vi "IMU Main.vi"() -> ()   [LabVIEW 2021]
doc: "This Continuous Measurement sample project is based on the Queued Message Handler template.\n\nThe Event Handling Loop generates messages based on user interface actions.\n\nThe Message Handling Loop processes messages generated by the Event Handling Loop, or by other messages. There are also Acquisition and Logging message handling loop subVIs, and a chart updating loop."
uses:
  Acquisition/IMU Data Queue.ctl
  IMU TimeDataStruct.ctl
  Acquisition/IMU Data Notifier.ctl
  Settings/Settings.ctl
  Acquisition/Hardware Configuration.ctl
  Settings/baudrates.ctl
  Logging/Logging Configuration.ctl
  controls/IMU UI Data.ctl
  controls/IMU UI State.ctl
  <vilib>/Platform/TimedLoop/XDataNode/timing_clust.ctl
  <vilib>/Platform/TimedLoop/XDataNode/nitl_modes.ctl
  <vilib>/Platform/TimedLoop/XDataNode/wakeup.ctl
  support/Message Queue/Enqueue Message (Single).vi
  support/Message Queue/Enqueue Message (Array).vi
  <vilib>/Utility/error.llb/Error Cluster From Error Code.vi
  <vilib>/ErrorRing/Error Ring.xnode
  <vilib>/platform/TimedLoop/XDataNode/XDataNode.xnode
  Acquisition/IMU Acquisition.lvlib
  Settings/IMU Settings.lvlib
  Logging/IMU Logging.lvlib
  support/User Event - Stop/IMU User Event - Stop.lvlib
  support/Message Queue/IMU Message Queue.lvlib
  Settings/Settings Dialog.vi
  Processing/IMU Processing.lvlib
  <vilib>/Platform/TimedLoop/XDataNode/XDNodeRunTimeDep.lvlib
  <vilib>/picture/3D Picture Control/NI_3D Picture Control.lvlib
  Processing/QuaternionLibrary/QuaternionLibrary.lvlib
panel:
  out "Quaternion":dbl[](array[numeric])
  out "IMU":refnum<vi>(3d-picture)
  in  "Enum 3":enum16{"None", "Disc", "Box", "STL"}(ring)=enum."Disc"
  in  "Frequency":i64
  in  "Data Queue Processing":T1
  in  "Data Notifier":T2
  in  "Data Queue Logging":T1
  in  "Settings":bool
  in  "Start":bool
  in  "Stop":bool
  out "Status":string
  in  "Exit":bool
  # "Continuous Measurement Data Logger"
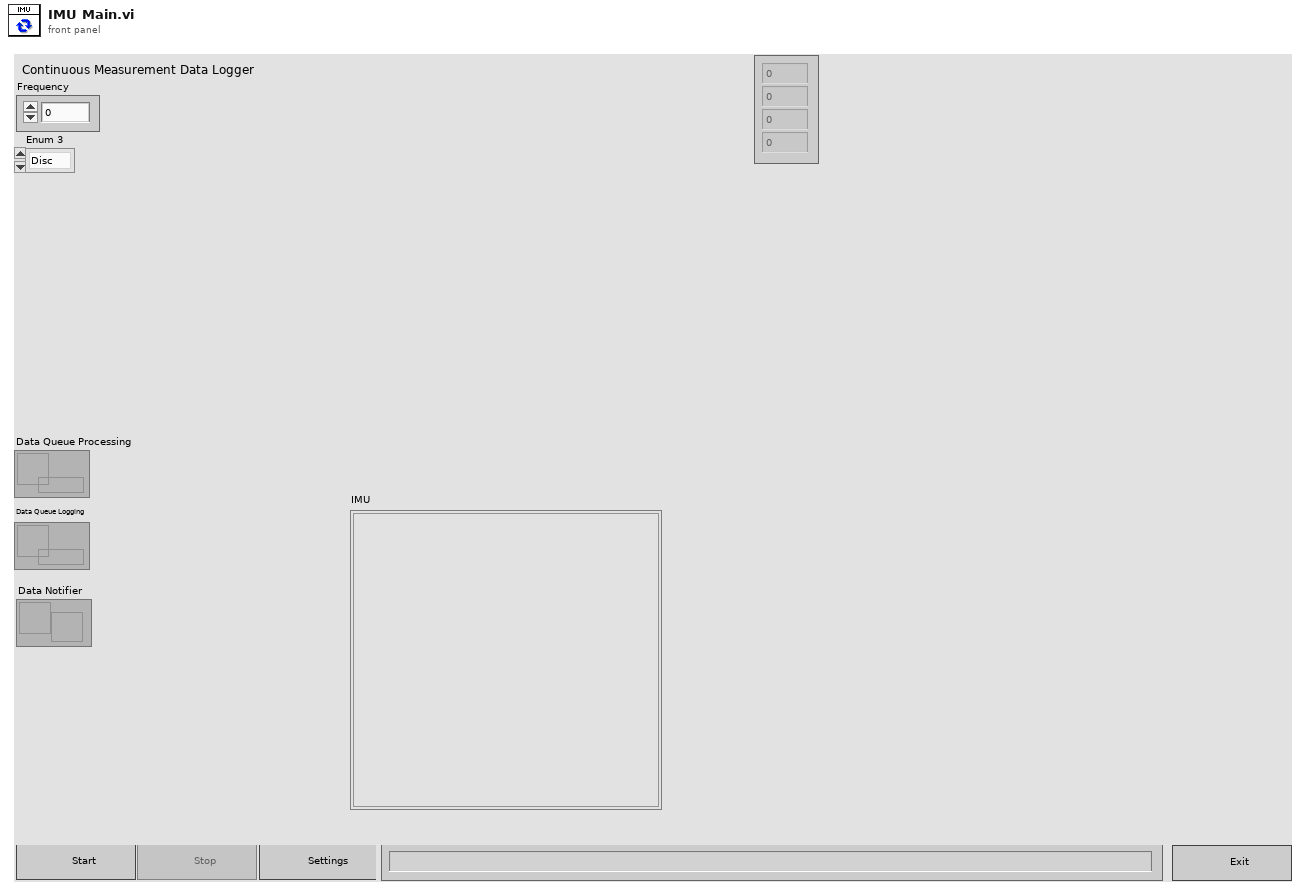
[diagram p1: front panel]
types:
  T1 = typedef "IMU Data Queue.ctl" = refnum<queue>
  T2 = typedef "IMU Data Notifier.ctl" = refnum<notifier>
  T3 = typedef "IMU TimeDataStruct.ctl" = cluster{string, dbl[]}
  T4 = typedef "IMU UI State.ctl" = enum16{"Idle", "Acquiring and Logging", "Waiting for Exit", "Waiting for Exit (Acq Stopped)", "Waiting for Exit (Log Stopped)", "Waiting for Stop", "Waiting for Stop (Acq Stopped)", "Waiting for Stop (Log Stopped)"}
  T5 = typedef "IMU UI Data.ctl" = cluster{"Start Ref":refnum<vi>, "Stop Ref":refnum<vi>, "Settings Ref":refnum<vi>, "Exit Ref":refnum<vi>, "Status Ref":refnum<vi>}
  T6 = typedef "IMU Settings.lvlib/Settings.ctl" = cluster{"Hardware Configuration":T7, "Logging Configuration":T9}
  T7 = typedef "IMU Acquisition.lvlib/Hardware Configuration.ctl" = cluster{"Port":refnum<visa-resource-name>, "Baudrate":T8}
  T8 = typedef "baudrates.ctl" = u16
  T9 = typedef "IMU Logging.lvlib/Logging Configuration.ctl" = cluster{"Log File Base Path":path, "TDMS File Reference":refnum<k34>, "Log Select":bool}
  T10 = typedef "IMU Message Queue.lvlib/All Message Queues.ctl" = cluster{"UI":refnum<queue>, "Acquisition":refnum<queue>, "Logging":refnum<queue>, "Processing":refnum<queue>}
  T11 = typedef "XDNodeRunTimeDep.lvlib/timing_clust.ctl" = cluster{"Expected End [f-1]":u64, "Actual End [f-1]":u64, "Finished Late? [f-1]":bool, "Expected End [i-1]":u64, "Actual End [i-1]":u64, "Finished Late? [i-1]":bool, "Expected Start [i]":u64, "Actual Start [i]":u64, "Expected Start [f]":u64, "Actual Start [f]":u64, "Source Name":string, "Structure Name":string, "Period":i64, "Deadline":i64, "Offset":i64, "Start":i64, "Priority":i32, "Timeout":i32, "Mode":T12, "Wakeup Reason":T13, "Error":errorcluster, "Source Type":string, "Secondary Source Type":string, "Global End Time":u64, "Global Start Time":u64, "Frame Duration":u64, "Iteration Duration":u64, "Assigned CPU":i32, "I/O Scan Engine Mode":u32}
  T12 = typedef "XDNodeRunTimeDep.lvlib/nitl_modes.ctl" = enum32{"No Change", "Process missed periods, maintain original phase", "Discard missed periods, maintain original phase", "Process missed periods, ignore original phase", "Discard missed periods, ignore original phase"}
  T13 = typedef "XDNodeRunTimeDep.lvlib/wakeup.ctl" = enum32{"Normal", "Aborted", "Asynchronous wakeup", "Timing source error", "Timed loop error", "Timeout"}
  T14 = cluster{"axis[0]":dbl, "axis[1]":dbl, "axis[2]":dbl}
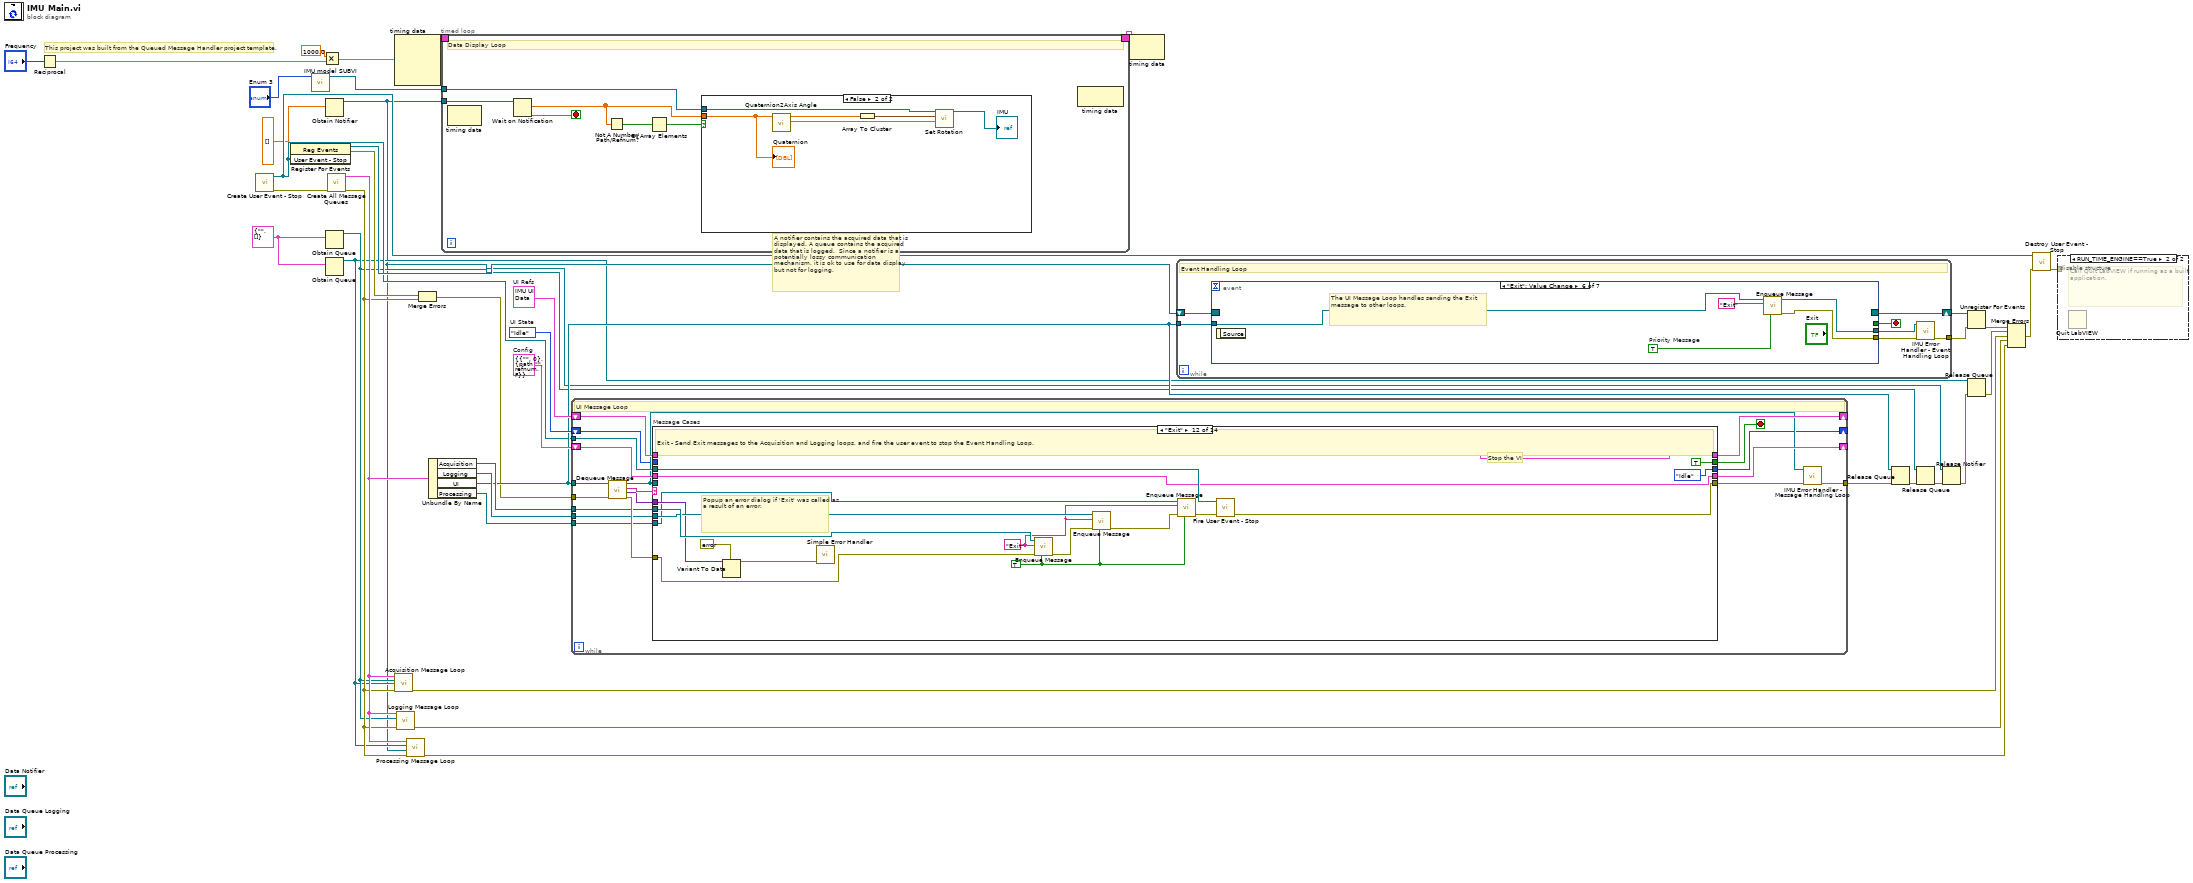
[diagram p0: block diagram]
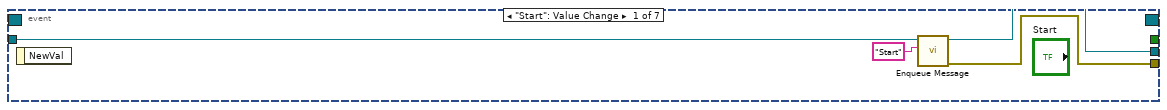
[diagram p4: hidden frame]
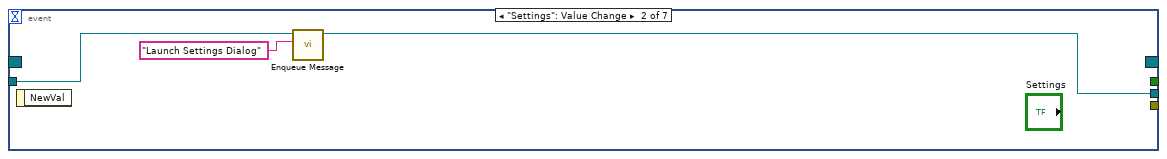
[diagram p5: hidden frame]
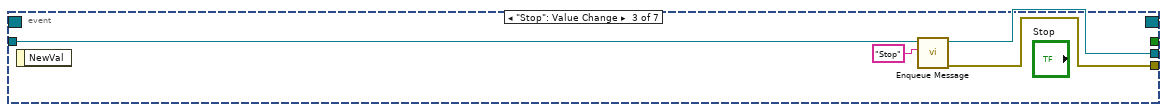
[diagram p6: hidden frame]
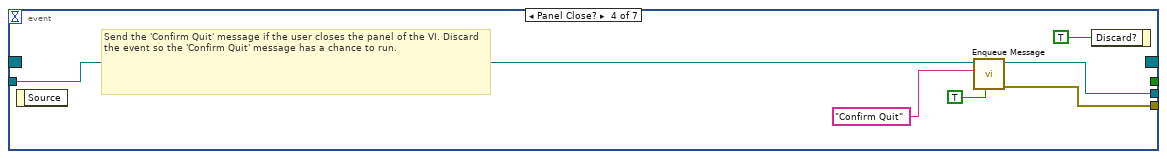
[diagram p7: hidden frame]
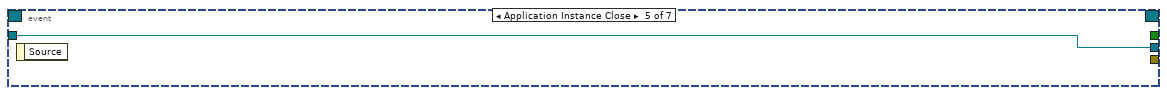
[diagram p8: hidden frame]
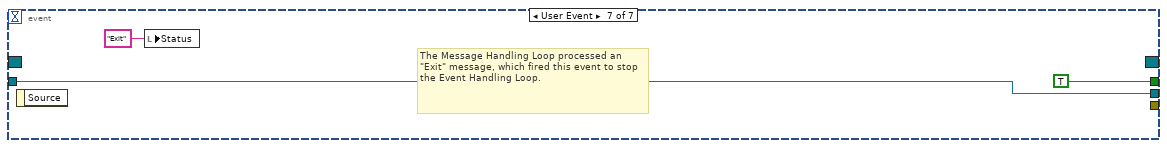
[diagram p9: hidden frame]
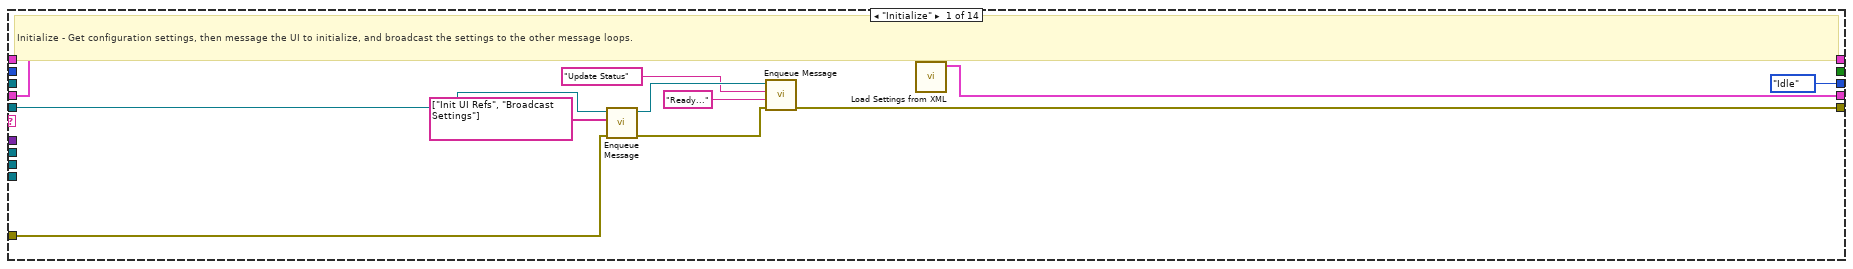
[diagram p10: hidden frame]
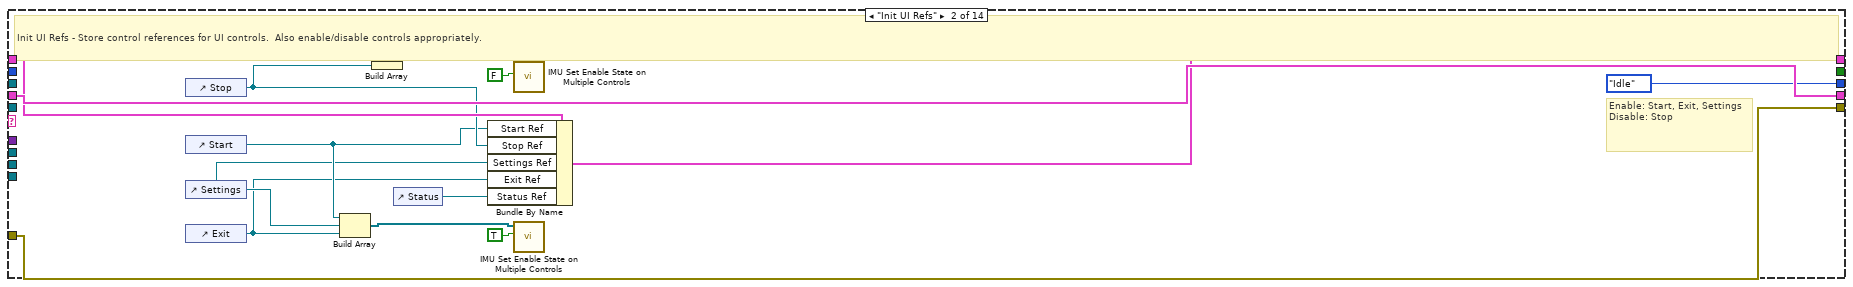
[diagram p11: hidden frame]
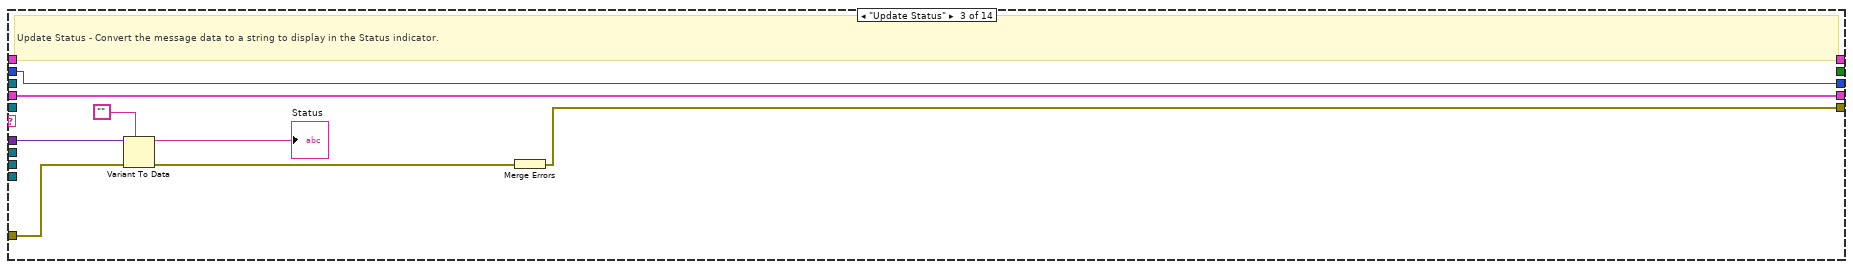
[diagram p12: hidden frame]
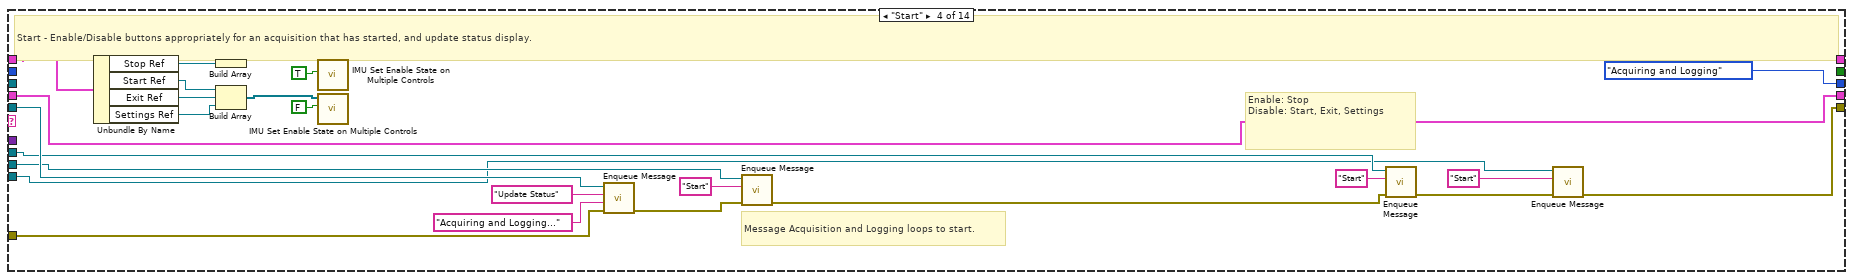
[diagram p13: hidden frame]
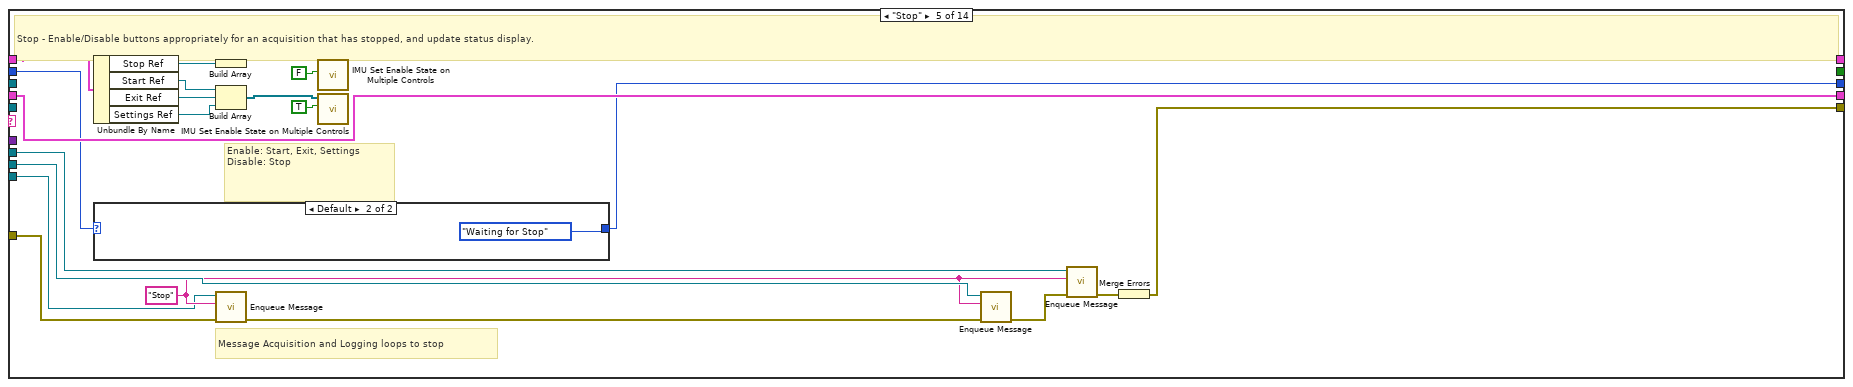
[diagram p14: hidden frame]
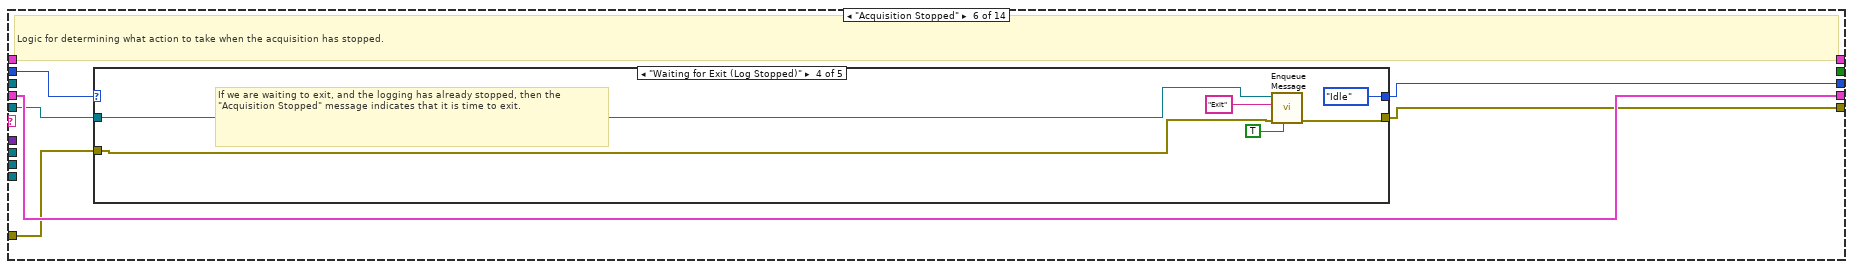
[diagram p16: hidden frame]
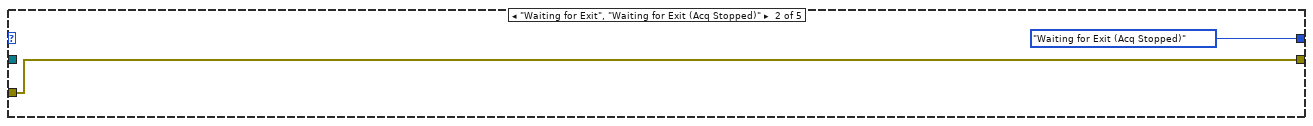
[diagram p18: hidden frame]
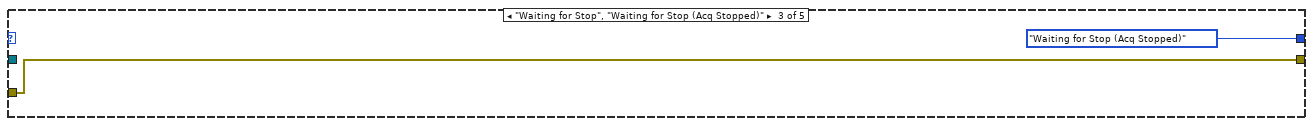
[diagram p19: hidden frame]
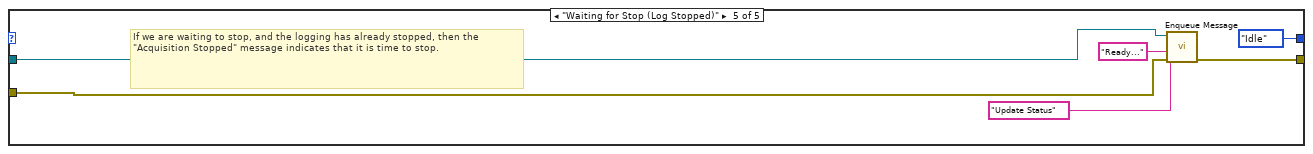
[diagram p20: hidden frame]
diagram:
  w19 = T3 {"", []}
  w29 = IMU_UI_State."Idle"  # UI State
  w32 = T5 {"Start Ref"=refnum, "Stop Ref"=refnum, "Settings Ref"=refnum, "Exit Ref"=refnum, "Status Ref"=refnum}  # UI Refs
  w35 = T6 {"Hardware Configuration"={"Port"="", "Baudrate"=0}, "Logging Configuration"={"Log File Base Path"=path "", "TDMS File Reference"=refnum, "Log Select"=FALSE}}  # Config
  # "This project was built from the Queued Message Handler project template."
  n1 = Reciprocal(x="Frequency") -> (1/x=w9:dbl)
  n2 = call "Create User Event - Stop.vi"() -> ("error out"=w37:errorcluster, "User Event - Stop"=w22:refnum<user-event>)  [unwired: 10 in]
  n3 = register-events(w22) -> (reference out=w23:refnum<event-registration>, error out=w20:errorcluster)  [unwired: 2 in]
  n4 = call "IMU model SUBVI.vi"("Enum 3"="Enum 3") -> ("SceneObject out"=w3:refnum<vi>)  [unwired: 10 in]
  n5 = Multiply(x=1000.0, y=w9) -> (x*y=w1:dbl)
  n6 = Obtain Queue(element data type=w19) -> (queue out=w14:refnum<queue>)  [unwired: 4 in, 2 out]
  n7 = Obtain Queue(element data type=w19) -> (queue out=w13:refnum<queue>)  [unwired: 4 in, 2 out]
  n8 = Obtain Notifier(notification data type=dbl[] []) -> (notifier out=w2:refnum<notifier>)  [unwired: 3 in, 2 out]
  n9 = call "Create All Message Queues.vi"("error in (no error)"=w37) -> ("error out"=w16:errorcluster, "Message Queues out"=w17:T10)  [unwired: 9 in]
  n10 = node-c288(w1) -> (w5:T11)  [unwired: 3 in]
  n11 = call "Acquisition Message Loop.vi"("Message Queues"=w17, "Data Queue Logging"=w14, "Data Queue Processing"=w13, "error in (no error)"=w16) -> ("error out"=w38:errorcluster)  [unwired: 11 in]
  n12 = call "Logging Message Loop.vi"("error in (no error)"=w16, "Data Queue"=w14, "Message Queues"=w17) -> ("error out"=w36:errorcluster)  [unwired: 8 in]
  n13 = call "Processing Message Loop.vi"("error in (no error)"=w16, "Data Notifier"=w2, "Data Queue"=w13, "Message Queues"=w17) -> ("error out"=w15:errorcluster)  [unwired: 7 in]
  n14 = Merge Errors(w20, w16) -> (w21:errorcluster)
  n15 = Unbundle By Name(w17) -> ("Acquisition"=w31:refnum<queue>, "Logging"=w30:refnum<queue>, "UI"=w27:refnum<queue>, "Processing"=w18:refnum<queue>)
  n16 = timed-loop "Data Display Loop" {
    timing: w5 -> [_]
    timing-out: [_] -> w4
    tunnel: w3 -> [w44]
    tunnel: w2 -> [w45]
    stop <- w46 stop-if-true
    # "A notifier contains the acquired data that is displayed. A queue contains the acquired data that is logged.  Since a notifier is a potentially lossy communication mechanism, it is ok to use for data display, but not for logging."
    # "Data Display Loop"
    n17 = node-c288() -> ()  [unwired: 1 in, 1 out]
    n18 = Wait on Notification(notifier=w45) -> (notification=w42:dbl[], error out=w46:errorcluster)  [unwired: 3 in, 2 out]
    n19 = Not A Number/Path/Refnum?(number/path/refnum=w42) -> (NaN/Path/Refnum?=w41:bool[])
    n20 = Or Array Elements(Boolean array=w41) -> (logical OR=w43:bool)
    n21 = case shown="False" w43 {
      tunnel: w42 -> [_ w52]
      tunnel: w44 -> [_ w48]
      frame True {
      }
      frame False {
        n22 = call <userlib>:"Quaternion2Axis Angle.vi"("quaternion"=w52) -> ("angle"=w51:sgl, "axis"=w50:dbl[])  [unwired: 8 in, 1 out]
        n23 = Array To Cluster(array=w50) -> (cluster=w49:T14)
        n24 = call <vilib>:"Set Rotation.vi"("Angle"=w51, "Axis"=w49, "Scene Object"=w48) -> ("Rotated Scene Object"=→"IMU":refnum<vi>)  [unwired: 7 in, 1 out]
        "Quaternion" <- w52
      }
    }
    n25 = node-c288() -> ()  [unwired: 1 in, 1 out]
  }
  n26 = while {
    tunnel: w27 -> [w67]
    tunnel: w22 -> [w72]
    shift-right: [w66] -> _
    shift-left: w35 -> [w65]
    shift-right: [w63] -> _
    shift-left: w32 -> [w64]
    tunnel: w31 -> [w62]
    tunnel: w30 -> [w61]
    shift-right: [w56] -> _
    shift-left: w29 -> [w57]
    tunnel: w21 -> [w71]
    tunnel: [w60] -> w40
    tunnel: w18 -> [w55]
    stop <- w73 stop-if-true
    # "UI Message Loop"
    n27 = call "Dequeue Message.vi"("error in (no error)"=w71, "Message Queue"=w67) -> ("error out"=w70:errorcluster, "Message Data"=w68:variant, "Message"=w69:string, "dup Message Queue"=w58:refnum<queue>)  [unwired: 6 in]
    n28 = case "Message Cases" shown="\"Exit\"" w69 {
      selector: w69 -> [_ _ _ _ _ _ _ _ _ _ _ _ _ w294]
      tunnel: w58 -> [w77 _ _ w133 _ w159 w184 _ w224 _ w245 _ _ _]
      tunnel: w70 -> [w76 w99 w107 w132 w136 w160 w185 w213 w226 w233 w244 w278 w292 _]
      tunnel: [w81 w99 w108 w110 w154 w157 w182 w218 w219 w236 w243 w285 w291 w293] -> w59
      tunnel: [_ _ _ _ _ _ _ _ _ _ _ TRUE _ _] -> w73
      tunnel: w68 -> [_ _ w106 _ _ _ _ _ _ w237 _ w276 _ _]
      tunnel: w72 -> [_ _ _ _ _ _ _ _ _ _ _ w286 _ _]
      tunnel: [w84 w98 w102 w131 w153 w163 w188 w216 w223 w241 w248 w284 w290 w297] -> w66
      tunnel: w65 -> [w85 w98 w102 w131 w153 w163 w188 w216 w227 w241 w248 w284 w290 w297]
      tunnel: w64 -> [w78 w97 w101 w128 w152 w162 w187 w212 w221 w240 w247 w283 w289 w296]
      tunnel: [w78 w95 w101 w128 w152 w162 w187 w212 w221 w240 w247 w283 w289 w296] -> w63
      tunnel: w62 -> [_ _ _ w115 w140 _ _ w211 _ _ _ w282 _ _]
      tunnel: w61 -> [_ _ _ w117 w143 _ _ w210 _ _ _ w281 _ _]
      tunnel: w57 -> [_ _ w100 _ w138 w161 w186 w209 w220 w235 w246 _ w288 w295]
      tunnel: [IMU_UI_State."Idle" ("UI State") IMU_UI_State."Idle" ("UI State") w100 IMU_UI_State."Acquiring and Logging" ("UI State") w139 w158 w183 w209 w220 w235 w242 IMU_UI_State."Idle" ("UI State") w288 w295] -> w56
      tunnel: w55 -> [_ _ _ w109 w134 _ _ _ _ _ _ w270 _ _]
      frame "Initialize" {
        # "Initialize - Get configuration settings, then message the UI to initialize, and broadcast the settings to the other message loops."
        n29 = call-poly "Enqueue Message.vi"("error in (no error)"=w76, "Message Array"=string[] ["Init UI Refs", "Broadcast Settings"], "Message Queue"=w77) -> ("error out"=w83:errorcluster, "dup Message Queue"=w82:refnum<queue>)  [unwired: 7 in]
        n30 = call-poly "Enqueue Message.vi"("error in (no error)"=w83, "Message Data"="Ready..." ("Ready..."), "Message"="Update Status", "Message Queue"=w82) -> ("error out"=w81:errorcluster)  [unwired: 6 in, 1 out]
        n31 = call "Load Settings from XML.vi"("Settings in"=w85) -> ("Settings out"=w84:T6)  [unwired: 9 in, 1 out]
      }
      frame "Init UI Refs" {
        # "Enable: Start, Exit, Settings\nDisable: Stop"
        # "Init UI Refs - Store control references for UI controls.  Also enable/disable controls appropriately."
        n32 = control-ref of="Stop"() -> (w90:refnum<vi>)
        n33 = control-ref of="Start"() -> (w89:refnum<vi>)
        n34 = control-ref of="Settings"() -> (w88:refnum<vi>)
        n35 = control-ref of="Exit"() -> (w87:refnum<vi>)
        n36 = Build Array(w89, w88, w87) -> (w93:refnum<vi>[])
        n37 = Build Array(w90) -> (w92:refnum<vi>[])
        n38 = control-ref of="Status"() -> (w96:refnum<vi>)
        n39 = Bundle By Name(cluster=w97, "Start Ref"=w89, "Stop Ref"=w90, "Settings Ref"=w88, "Exit Ref"=w87, "Status Ref"=w96) -> (w95:T5)
        n40 = call "IMU Set Enable State on Multiple Controls.vi"("Enable?"=FALSE, "Controls"=w92) -> ()  [unwired: 10 in]
        n41 = call "IMU Set Enable State on Multiple Controls.vi"("Enable?"=TRUE, "Controls"=w93) -> ()  [unwired: 10 in]
      }
      frame "Update Status" {
        # "Update Status - Convert the message data to a string to display in the Status indicator."
        n42 = Variant To Data(error in=w107, type="", Variant=w106) -> (data=→"Status":string, error out=w104:errorcluster)
        n43 = Merge Errors(w104) -> (w108:errorcluster)
      }
      frame "Start" {
        # "Message Acquisition and Logging loops to start."
        # "Enable: Stop\nDisable: Start, Exit, Settings"
        # "Start - Enable/Disable buttons appropriately for an acquisition that has started, and update status display."
        n44 = Unbundle By Name(w128) -> ("Stop Ref"=w123:refnum<vi>, "Start Ref"=w122:refnum<vi>, "Exit Ref"=w121:refnum<vi>, "Settings Ref"=w120:refnum<vi>)
        n45 = Build Array(w123) -> (w125:refnum<vi>[])
        n46 = Build Array(w122, w121, w120) -> (w126:refnum<vi>[])
        n47 = call "IMU Set Enable State on Multiple Controls.vi"("Enable?"=TRUE, "Controls"=w125) -> ()  [unwired: 10 in]
        n48 = call "IMU Set Enable State on Multiple Controls.vi"("Enable?"=FALSE, "Controls"=w126) -> ()  [unwired: 10 in]
        n49 = call-poly "Enqueue Message.vi"("error in (no error)"=w132, "Message Data"="Acquiring and Logging..." ("Acquiring and Logging..."), "Message"="Update Status", "Message Queue"=w133) -> ("error out"=w119:errorcluster)  [unwired: 6 in, 1 out]
        n50 = call-poly "Enqueue Message.vi"("error in (no error)"=w119, "Message"="Start", "Message Queue"=w117) -> ("error out"=w116:errorcluster)  [unwired: 7 in, 1 out]
        n51 = call-poly "Enqueue Message.vi"("error in (no error)"=w116, "Message"="Start", "Message Queue"=w115) -> ("error out"=w111:errorcluster)  [unwired: 7 in, 1 out]
        n52 = call-poly "Enqueue Message.vi"("error in (no error)"=w111, "Message"="Start", "Message Queue"=w109) -> ("error out"=w110:errorcluster)  [unwired: 7 in, 1 out]
      }
      frame "Stop" {
        w135 = "Stop" ("Message")
        # "Message Acquisition and Logging loops to stop"
        # "Enable: Start, Exit, Settings\nDisable: Stop"
        # "Stop - Enable/Disable buttons appropriately for an acquisition that has stopped, and update status display."
        n53 = Unbundle By Name(w152) -> ("Stop Ref"=w147:refnum<vi>, "Start Ref"=w146:refnum<vi>, "Exit Ref"=w145:refnum<vi>, "Settings Ref"=w144:refnum<vi>)
        n54 = case shown="Default" w138 {
          selector: w138 -> [w155 _]
          tunnel: [w155 IMU_UI_State."Waiting for Stop" ("UI State")] -> w139
          frame "Waiting for Exit" {
          }
          frame Default {
          }
        }
        n55 = Build Array(w147) -> (w149:refnum<vi>[])
        n56 = Build Array(w146, w145, w144) -> (w150:refnum<vi>[])
        n57 = call-poly "Enqueue Message.vi"("error in (no error)"=w136, "Message"=w135, "Message Queue"=w134) -> ("error out"=w137:errorcluster)  [unwired: 7 in, 1 out]
        n58 = call "IMU Set Enable State on Multiple Controls.vi"("Enable?"=FALSE, "Controls"=w149) -> ()  [unwired: 10 in]
        n59 = call "IMU Set Enable State on Multiple Controls.vi"("Enable?"=TRUE, "Controls"=w150) -> ()  [unwired: 10 in]
        n60 = call-poly "Enqueue Message.vi"("error in (no error)"=w137, "Message"=w135, "Message Queue"=w143) -> ("error out"=w142:errorcluster)  [unwired: 7 in, 1 out]
        n61 = call-poly "Enqueue Message.vi"("error in (no error)"=w142, "Message"=w135, "Message Queue"=w140) -> ("error out"=w141:errorcluster)  [unwired: 7 in, 1 out]
        n62 = Merge Errors(w141) -> (w154:errorcluster)
      }
      frame "Acquisition Stopped" {
        # "Logic for determining what action to take when the acquisition has stopped."
        n63 = case shown="\"Waiting for Exit (Log Stopped)\"" w161 {
          selector: w161 -> [w165 _ _ _ _]
          tunnel: w160 -> [w164 w167 w169 w175 w181]
          tunnel: w159 -> [_ _ _ w173 w178]
          tunnel: [w165 IMU_UI_State."Waiting for Exit (Acq Stopped)" ("UI State") IMU_UI_State."Waiting for Stop (Acq Stopped)" ("UI State") IMU_UI_State."Idle" ("UI State") IMU_UI_State."Idle" ("UI State")] -> w158
          tunnel: [w164 w167 w169 w174 w179] -> w157
          frame Default {
          }
          frame "Waiting for Exit", "Waiting for Exit (Acq Stopped)" {
          }
          frame "Waiting for Stop", "Waiting for Stop (Acq Stopped)" {
          }
          frame "Waiting for Exit (Log Stopped)" {
            # "If we are waiting to exit, and the logging has already stopped, then the \"Acquisition Stopped\" message indicates that it is time to exit."
            n64 = call-poly "Enqueue Message.vi"("Priority Message? (F)"=TRUE, "error in (no error)"=w175, "Message"="Exit", "Message Queue"=w173) -> ("error out"=w174:errorcluster)  [unwired: 6 in, 1 out]
          }
          frame "Waiting for Stop (Log Stopped)" {
            # "If we are waiting to stop, and the logging has already stopped, then the \"Acquisition Stopped\" message indicates that it is time to stop."
            n65 = call-poly "Enqueue Message.vi"("error in (no error)"=w181, "Message Data"="Ready..." ("Ready..."), "Message"="Update Status", "Message Queue"=w178) -> ("error out"=w179:errorcluster)  [unwired: 6 in, 1 out]
          }
        }
      }
      frame "Logging Stopped" {
        # "Logic for determining what action to take when the logging has stopped."
        n66 = case shown="\"Waiting for Stop (Acq Stopped)\"" w186 {
          selector: w186 -> [w190 _ _ _ _]
          tunnel: w185 -> [w189 w192 w194 w200 w203]
          tunnel: w184 -> [_ _ _ w198 w202]
          tunnel: [w190 IMU_UI_State."Waiting for Exit (Log Stopped)" ("UI State") IMU_UI_State."Waiting for Stop (Log Stopped)" ("UI State") IMU_UI_State."Idle" ("UI State") IMU_UI_State."Idle" ("UI State")] -> w183
          tunnel: [w189 w192 w194 w199 w201] -> w182
          frame Default {
          }
          frame "Waiting for Exit", "Waiting for Exit (Log Stopped)" {
          }
          frame "Waiting for Stop", "Waiting for Stop (Log Stopped)" {
          }
          frame "Waiting for Exit (Acq Stopped)" {
            # "If we are waiting to exit, and the acquisition has already stopped, then the \"Logging Stopped\" message indicates that it is time to exit."
            n67 = call-poly "Enqueue Message.vi"("Priority Message? (F)"=TRUE, "error in (no error)"=w200, "Message"="Exit", "Message Queue"=w198) -> ("error out"=w199:errorcluster)  [unwired: 6 in, 1 out]
          }
          frame "Waiting for Stop (Acq Stopped)" {
            # "If we are waiting to stop, and the acquisition has already stopped, then the \"Logging Stopped\" message indicates that it is time to stop."
            n68 = call-poly "Enqueue Message.vi"("error in (no error)"=w203, "Message Data"="Ready..." ("Ready..."), "Message"="Update Status", "Message Queue"=w202) -> ("error out"=w201:errorcluster)  [unwired: 6 in, 1 out]
          }
        }
      }
      frame "Broadcast settings" {
        w208 = "Update Settings" ("Message")
        # "Broadcast settings - Send the 'Update Settings' message to the Logging and Acquisition message loops."
        n69 = Unbundle By Name(w216) -> ("Hardware Configuration"=w215:T7, "Logging Configuration"=w214:T9)
        n70 = call-poly "Enqueue Message.vi"("Message Data"=w215, "Message"=w208, "Message Queue"=w211) -> ("error out"=w217:errorcluster)  [unwired: 7 in, 1 out]
        n71 = call-poly "Enqueue Message.vi"("error in (no error)"=w217, "Message Data"=w214, "Message"=w208, "Message Queue"=w210) -> ("error out"=w207:errorcluster)  [unwired: 6 in, 1 out]
        n72 = Merge Errors(w207, w213) -> (w218:errorcluster)
      }
      frame "Launch Settings Dialog" {
        # "Launch Settings Dialog - Launch the Settings Dialog when the user clicks the 'Settings' button."
        n73 = call-by-ref "?"("error in (no error)"=w226, "Settings in"=w227) -> ("error out"=w222:errorcluster, "Cancelled?"=w225:bool, "Settings out"=w223:T6)  [unwired: 8 in, 3 out]
        n74 = case shown="False" w225 {
          tunnel: w224 -> [w231 _]
          tunnel: w222 -> [w230 w232]
          tunnel: [w229 w232] -> w219
          frame False {
            n75 = call-poly "Enqueue Message.vi"("error in (no error)"=w230, "Message"="Broadcast Settings", "Message Queue"=w231) -> ("error out"=w229:errorcluster)  [unwired: 7 in, 1 out]
          }
          frame True {
          }
        }
      }
      frame "Error" {
        # "Error - Display an error dialog. This message is sent by the \"Error Handler\" VIs at the end of other loops in this application."
        n76 = Variant To Data(error in=w233, type=errorcluster {"status"=FALSE, "code"=0, "source"=""} ("error constant"), Variant=w237) -> (data=w234:errorcluster, error out=w238:errorcluster)
        n77 = call <vilib>:"Simple Error Handler.vi"("error in (no error)"=w234) -> ()  [unwired: 4 in, 5 out]
        n78 = Merge Errors(w238) -> (w236:errorcluster)
      }
      frame "Confirm Quit" {
        # "Confirm Quit - Message that can confirm whether or not the user wants to exit the application."
        n79 = case shown="Default" w246 {
          tunnel: w245 -> [w254 w258]
          tunnel: w244 -> [w253 w257]
          tunnel: [w252 w256] -> w243
          tunnel: [IMU_UI_State."Idle" ("UI State") w255] -> w242
          frame Default {
            # "If 'Confirm Quit' comes in while the system is idle, there is no need for a confirmation message."
            n80 = call-poly "Enqueue Message.vi"("Priority Message? (F)"=TRUE, "error in (no error)"=w253, "Message"="Exit", "Message Queue"=w254) -> ("error out"=w252:errorcluster)  [unwired: 6 in, 1 out]
          }
          frame "Acquiring and Logging" {
            n81 = Two Button Dialog(message="Are you sure you want to quit while the acquisition is running?" ("Confirm Quit Message"), 1:"No" ("No"), 2:"Yes" ("Yes")) -> (T button?=w259:bool)
            n82 = case shown="True" w259 {
              tunnel: w258 -> [_ w268]
              tunnel: w257 -> [w264 w269]
              tunnel: [w264 w267] -> w256
              tunnel: [IMU_UI_State."Acquiring and Logging" ("UI State") IMU_UI_State."Waiting for Exit" ("UI State")] -> w255
              frame False {
                # "User did not want to quit."
              }
              frame True {
                n83 = call-poly "Enqueue Message.vi"("error in (no error)"=w269, "Message"="Stop", "Message Queue"=w268) -> ("error out"=w267:errorcluster)  [unwired: 7 in, 1 out]
              }
            }
          }
        }
      }
      frame "Exit" {
        w271 = TRUE ("Priority Message? (F)")
        w274 = "Exit" ("Message")
        # "Popup an error dialog if 'Exit' was called as a result of an error."
        # "Stop the VI"
        # "Exit - Send Exit messages to the Acquisition and Logging loops, and fire the user event to stop the Event Handling Loop."
        n84 = Variant To Data(type=errorcluster {"status"=FALSE, "code"=0, "source"=""} ("error constant"), Variant=w276) -> (data=w275:errorcluster)  [unwired: 1 in, 1 out]
        n85 = call <vilib>:"Simple Error Handler.vi"("error in (no error)"=w275) -> ()  [unwired: 4 in, 5 out]
        n86 = call-poly "Enqueue Message.vi"("Priority Message? (F)"=w271, "error in (no error)"=w278, "Message"=w274, "Message Queue"=w282) -> ("error out"=w279:errorcluster)  [unwired: 6 in, 1 out]
        n87 = call-poly "Enqueue Message.vi"("Priority Message? (F)"=w271, "error in (no error)"=w279, "Message"=w274, "Message Queue"=w281) -> ("error out"=w273:errorcluster)  [unwired: 6 in, 1 out]
        n88 = call-poly "Enqueue Message.vi"("Priority Message? (F)"=w271, "error in (no error)"=w273, "Message"=w274, "Message Queue"=w270) -> ("error out"=w272:errorcluster)  [unwired: 6 in, 1 out]
        n89 = call "Fire User Event - Stop.vi"("error in (no error)"=w272, "User Event - Stop"=w286) -> ("error out"=w285:errorcluster)  [unwired: 9 in]
      }
      frame "---Copy This Frame---" {
        # "Duplicate this frame when creating new messages.  Change this comment in the duplicated frame to describe this message."
        n90 = Merge Errors(w292) -> (w291:errorcluster)
      }
      frame Default {
        # "'Default' case only runs if there is a message that isn't defined in any of the other cases.  Output a programming error."
        n91 = xnode "Error Ring"("parameter 0"=w294) -> ("error out"=w293:errorcluster)
      }
    }
    n92 = call "IMU Error Handler - Message Handling Loop.vi"("error in (no error)"=w59, "Message Queue"=w58) -> ("dup error in"=w60:errorcluster)  [unwired: 8 in, 1 out]
  }
  n93 = node-c288(w4) -> ()  [unwired: 1 out]
  n94 = while {
    tunnel: w27 -> [w310]
    tunnel: [w307] -> w39
    shift-right: [w309] -> w33
    shift-left: w23 -> [w311]
    stop <- w308 stop-if-true
    # "Event Handling Loop"
    n95 = event shown="[5] \"Exit\": Value Change" {
      selector: w311 -> [_ _ _ _ _ _ _]
      dyn-events: [_ _ _ _ _ _ _] -> w309
      timeout: _ -> [_ _ _ _ _ _ _]
      tunnel: [_ _ _ _ _ _ TRUE ("Discard?")] -> w308
      tunnel: w310 -> [w315 w317 w321 w326 w329 w331 w335]
      tunnel: [w313 _ w320 w324 _ w334 _] -> w306
      tunnel: [w312 w316 w319 w325 w329 w330 w335] -> w305
      event "Start": Value Change {
        n96 = event-data() -> ()  [unwired: 1 in, 1 out]
        n97 = call-poly "Enqueue Message.vi"("Message"="Start", "Message Queue"=w315) -> ("error out"=w313:errorcluster, "dup Message Queue"=w312:refnum<queue>)  [unwired: 8 in]
      }
      event "Settings": Value Change {
        n98 = event-data() -> ()  [unwired: 1 in, 1 out]
        n99 = call-poly "Enqueue Message.vi"("Message"="Launch Settings Dialog", "Message Queue"=w317) -> ("dup Message Queue"=w316:refnum<queue>)  [unwired: 8 in, 1 out]
      }
      event "Stop": Value Change {
        n100 = event-data() -> ()  [unwired: 1 in, 1 out]
        n101 = call-poly "Enqueue Message.vi"("Message"="Stop", "Message Queue"=w321) -> ("error out"=w320:errorcluster, "dup Message Queue"=w319:refnum<queue>)  [unwired: 8 in]
      }
      event Panel Close? {
        # "Send the 'Confirm Quit' message if the user closes the panel of the VI. Discard the event so the 'Confirm Quit' message has a chance to run."
        n102 = event-data() -> ()  [unwired: 1 in, 1 out]
        n103 = call-poly "Enqueue Message.vi"("Priority Message? (F)"=TRUE, "Message"="Confirm Quit", "Message Queue"=w326) -> ("error out"=w324:errorcluster, "dup Message Queue"=w325:refnum<queue>)  [unwired: 7 in]
        n104 = event-data("Discard?"=TRUE) -> ()  [unwired: 1 in, 1 out]
      }
      event Application Instance Close {
        n105 = event-data() -> ()  [unwired: 1 in, 1 out]
      }
      event "Exit": Value Change {
        w332 = TRUE  # Priority Message
        # "The UI Message Loop handles sending the Exit message to other loops."
        n106 = event-data() -> ()  [unwired: 1 in, 1 out]
        n107 = call-poly "Enqueue Message.vi"("Priority Message? (F)"=w332, "Message"="Exit", "Message Queue"=w331) -> ("error out"=w334:errorcluster, "dup Message Queue"=w330:refnum<queue>)  [unwired: 7 in]
      }
      event User Event {
        # "The Message Handling Loop processed an \"Exit\" message, which fired this event to stop the Event Handling Loop."
        n108 = event-data() -> ()  [unwired: 1 in, 1 out]
        n109 = local write "Status"("Exit" ("Exit String")) -> ()
      }
    }
    n110 = call "IMU Error Handler - Event Handling Loop.vi"("error in (no error)"=w306, "Message Queue"=w305) -> ("dup error in"=w307:errorcluster)  [unwired: 8 in, 1 out]
  }
  n111 = Release Queue(queue=w27, error in (no error)=w40) -> (error out=w25:errorcluster)  [unwired: 1 in, 2 out]
  n112 = Release Queue(queue=w14, error in (no error)=w25) -> (error out=w24:errorcluster)  [unwired: 1 in, 2 out]
  n113 = Release Notifier(notifier=w2, error in (no error)=w24) -> (error out=w12:errorcluster)  [unwired: 1 in, 2 out]
  n114 = Unregister For Events(event registration refnum=w33, error in=w39) -> (error out=w34:errorcluster)
  n115 = Release Queue(queue=w13, error in (no error)=w12) -> (error out=w11:errorcluster)  [unwired: 1 in, 2 out]
  n116 = Merge Errors(w34, w11, w38, w36, w15) -> (w28:errorcluster)
  n117 = call "Destroy User Event - Stop.vi"("error in (no error)"=w28, "User Event - Stop"=w22) -> ("error out"=w26:errorcluster)  [unwired: 9 in]
  n118 = disable-structure shown="RUN_TIME_ENGINE==True" {
    disable-tunnel: w26 -> [_ _]
    frame condition #0 (active) {
    }
    frame condition #1 {
      # "Call Quit LabVIEW if running as a built application."
      n119 = Quit LabVIEW() -> ()  [unwired: 1 in]
    }
  }
